vi "Plate Configuration(subVi).vi"(4 "출력 클러스터 2":T1, 5 "all rows":string[][](array[string])=[["", "Well", "Fluor", "Target", "Content", "Sample", "Cq", "SQ"], ["", "A01", "SYBR", "Fos", "Unkn", "Fl1", "23.40", ""], ["", "A02", "SYBR", "Fos", "Unkn", "Fl1", "23.24", ""], ["", "A03", "SYBR", "Fos", "Unkn", "Fl2", "23.55", ""], ["", "A04", "SYBR", "Fos", "Unkn", "Fl2", "23.53", ""], ["", "A05", "SYBR", "Fos", "Unkn", "Fl3", "23.38", ""], ["", "A06", "SYBR", "Fos", "Unkn", "Fl3", "23.50", ""], ["", "A07", "SYBR", "Fos", "Unkn", "Pfl1", "22.43", ""], ["", "A08", "SYBR", "Fos", "Unkn", "Pfl1", "22.94", ""], ["", "A09", "SYBR", "Fos", "Unkn", "Pfl2", "21.10", ""], ["", "A10", "SYBR", "Fos", "Unkn", "Pfl2", "21.46", ""], ["", "A11", "SYBR", "Fos", "Unkn", "Pfl3", "22.49", ""], ["", "A12", "SYBR", "Fos", "Unkn", "Pfl3", "22.89", ""], ["", "B01", "SYBR", "Arc", "Unkn", "Fl1", "32.28", ""], ["", "B02", "SYBR", "Arc", "Unkn", "Fl1", "32.59", ""], ["", "B03", "SYBR", "Arc", "Unkn", "Fl2", "32.93", ""], ["", "B04", "SYBR", "Arc", "Unkn", "Fl2", "32.78", ""], ["", "B05", "SYBR", "Arc", "Unkn", "Fl3", "32.38", ""], ["", "B06", "SYBR", "Arc", "Unkn", "Fl3", "32.35", ""], ["", "B07", "SYBR", "Arc", "Unkn", "Pfl1", "30.44", ""], ["", "B08", "SYBR", "Arc", "Unkn", "Pfl1", "30.58", ""], ["", "B09", "SYBR", "Arc", "Unkn", "Pfl2", "30.07", ""], ["", "B10", "SYBR", "Arc", "Unkn", "Pfl2", "30.20", ""], ["", "B11", "SYBR", "Arc", "Unkn", "Pfl3", "30.38", ""], ["", "B12", "SYBR", "Arc", "Unkn", "Pfl3", "30.04", ""], ["", "C01", "SYBR", "Jun", "Unkn", "Fl1", "25.27", ""], ["", "C02", "SYBR", "Jun", "Unkn", "Fl1", "24.72", ""], ["", "C03", "SYBR", "Jun", "Unkn", "Fl2", "25.47", ""], ["", "C04", "SYBR", "Jun", "Unkn", "Fl2", "25.79", ""], ["", "C05", "SYBR", "Jun", "Unkn", "Fl3", "25.27", ""], ["", "C06", "SYBR", "Jun", "Unkn", "Fl3", "25.52", ""], ["", "C07", "SYBR", "Jun", "Unkn", "Pfl1", "23.53", ""], ["", "C08", "SYBR", "Jun", "Unkn", "Pfl1", "23.37", ""], ["", "C09", "SYBR", "Jun", "Unkn", "Pfl2", "21.29", ""], ["", "C10", "SYBR", "Jun", "Unkn", "Pfl2", "38.35", ""], ["", "C11", "SYBR", "Jun", "Unkn", "Pfl3", "23.20", ""], ["", "C12", "SYBR", "Jun", "Unkn", "Pfl3", "23.23", ""], ["", "D01", "SYBR", "JunB", "Unkn", "Fl1", "26.08", ""], ["", "D02", "SYBR", "JunB", "Unkn", "Fl1", "26.09", ""], ["", "D03", "SYBR", "JunB", "Unkn", "Fl2", "27.02", ""], ["", "D04", "SYBR", "JunB", "Unkn", "Fl2", "27.08", ""], ["", "D05", "SYBR", "JunB", "Unkn", "Fl3", "26.91", ""], ["", "D06", "SYBR", "JunB", "Unkn", "Fl3", "26.93", ""], ["", "D07", "SYBR", "JunB", "Unkn", "Pfl1", "25.32", ""], ["", "D08", "SYBR", "JunB", "Unkn", "Pfl1", "25.12", ""], ["", "D09", "SYBR", "JunB", "Unkn", "Pfl2", "24.28", ""], ["", "D10", "SYBR", "JunB", "Unkn", "Pfl2", "24.21", ""], ["", "D11", "SYBR", "JunB", "Unkn", "Pfl3", "25.01", ""], ["", "D12", "SYBR", "JunB", "Unkn", "Pfl3", "25.38", ""], ["", "E01", "SYBR", "Ctgf", "Unkn", "Fl1", "27.57", ""], ["", "E02", "SYBR", "Ctgf", "Unkn", "Fl1", "27.52", ""], ["", "E03", "SYBR", "Ctgf", "Unkn", "Fl2", "28.24", ""], ["", "E04", "SYBR", "Ctgf", "Unkn", "Fl2", "28.02", ""], ["", "E05", "SYBR", "Ctgf", "Unkn", "Fl3", "28.10", ""], ["", "E06", "SYBR", "Ctgf", "Unkn", "Fl3", "27.90", ""], ["", "E07", "SYBR", "Ctgf", "Unkn", "Pfl1", "25.17", ""], ["", "E08", "SYBR", "Ctgf", "Unkn", "Pfl1", "25.51", ""], ["", "E09", "SYBR", "Ctgf", "Unkn", "Pfl2", "25.49", ""], ["", "E10", "SYBR", "Ctgf", "Unkn", "Pfl2", "25.43", ""], ["", "E11", "SYBR", "Ctgf", "Unkn", "Pfl3", "25.45", ""], ["", "E12", "SYBR", "Ctgf", "Unkn", "Pfl3", "25.45", ""], ["", "F01", "SYBR", "Nr4a1", "Unkn", "Fl1", "25.09", ""], ["", "F02", "SYBR", "Nr4a1", "Unkn", "Fl1", "25.24", ""], ["", "F03", "SYBR", "Nr4a1", "Unkn", "Fl2", "26.15", ""], ["", "F04", "SYBR", "Nr4a1", "Unkn", "Fl2", "26.01", ""], ["", "F05", "SYBR", "Nr4a1", "Unkn", "Fl3", "26.17", ""], ["", "F06", "SYBR", "Nr4a1", "Unkn", "Fl3", "26.29", ""], ["", "F07", "SYBR", "Nr4a1", "Unkn", "Pfl1", "24.23", ""], ["", "F08", "SYBR", "Nr4a1", "Unkn", "Pfl1", "24.26", ""], ["", "F09", "SYBR", "Nr4a1", "Unkn", "Pfl2", "23.05", ""], ["", "F10", "SYBR", "Nr4a1", "Unkn", "Pfl2", "23.08", ""], ["", "F11", "SYBR", "Nr4a1", "Unkn", "Pfl3", "24.02", ""], ["", "F12", "SYBR", "Nr4a1", "Unkn", "Pfl3", "24.04", ""], ["", "G01", "SYBR", "Egr1", "Unkn", "Fl1", "26.85", ""], ["", "G02", "SYBR", "Egr1", "Unkn", "Fl1", "26.59", ""], ["", "G03", "SYBR", "Egr1", "Unkn", "Fl2", "27.75", ""], ["", "G04", "SYBR", "Egr1", "Unkn", "Fl2", "27.76", ""], ["", "G05", "SYBR", "Egr1", "Unkn", "Fl3", "27.92", ""], ["", "G06", "SYBR", "Egr1", "Unkn", "Fl3", "28.27", ""], ["", "G07", "SYBR", "Egr1", "Unkn", "Pfl1", "25.19", ""], ["", "G08", "SYBR", "Egr1", "Unkn", "Pfl1", "24.90", ""], ["", "G09", "SYBR", "Egr1", "Unkn", "Pfl2", "23.36", ""], ["", "G10", "SYBR", "Egr1", "Unkn", "Pfl2", "23.81", ""], ["", "G11", "SYBR", "Egr1", "Unkn", "Pfl3", "24.67", ""], ["", "G12", "SYBR", "Egr1", "Unkn", "Pfl3", "24.81", ""], ["", "H01", "SYBR", "beta-Actin", "Unkn", "Fl1", "22.22", ""], ["", "H02", "SYBR", "beta-Actin", "Unkn", "Fl1", "22.27", ""], ["", "H03", "SYBR", "beta-Actin", "Unkn", "Fl2", "22.94", ""], ["", "H04", "SYBR", "beta-Actin", "Unkn", "Fl2", "22.82", ""], ["", "H05", "SYBR", "beta-Actin", "Unkn", "Fl3", "23.04", ""], ["", "H06", "SYBR", "beta-Actin", "Unkn", "Fl3", "22.72", ""], ["", "H07", "SYBR", "beta-Actin", "Unkn", "Pfl1", "22.09", ""], ["", "H08", "SYBR", "beta-Actin", "Unkn", "Pfl1", "22.09", ""], ["", "H09", "SYBR", "beta-Actin", "Unkn", "Pfl2", "21.57", ""], ["", "H10", "SYBR", "beta-Actin", "Unkn", "Pfl2", "21.16", ""], ["", "H11", "SYBR", "beta-Actin", "Unkn", "Pfl3", "21.80", ""], ["", "H12", "SYBR", "beta-Actin", "Unkn", "Pfl3", "21.93", ""]] caption="모든 행", 6 "RowLabel":T3(array[cluster])=[{"RowNames"="A", "Label"=enum."Target Ch"}, {"RowNames"="B", "Label"=enum."Target Ch"}, {"RowNames"="C", "Label"=enum."Target Ch"}, {"RowNames"="D", "Label"=enum."Target Ch"}, {"RowNames"="E", "Label"=enum."Target Ch"}, {"RowNames"="F", "Label"=enum."Target Ch"}, {"RowNames"="G", "Label"=enum."Target Ch"}, {"RowNames"="H", "Label"=enum."Internal Ctrl"}], 7 "ColLabel":T2(array[cluster])=[{"ColNames"="01", "Label"=enum."11"}, {"ColNames"="02", "Label"=enum."11"}, {"ColNames"="03", "Label"=enum."12"}, {"ColNames"="04", "Label"=enum."12"}, {"ColNames"="05", "Label"=enum."13"}, {"ColNames"="06", "Label"=enum."13"}, {"ColNames"="07", "Label"=enum."13"}, {"ColNames"="08", "Label"=enum."13"}, {"ColNames"="09", "Label"=enum."13"}, {"ColNames"="10", "Label"=enum."13"}, {"ColNames"="11", "Label"=enum."13"}, {"ColNames"="12", "Label"=enum."13"}]) -> (0 "출력 클러스터":T1, 1 "RowHdrs":string[](array[string]), 2 "Internal Ctrl":string[][](array[string]), 3 "Target Gene":string[][][](array[string]))   [LabVIEW 2015]
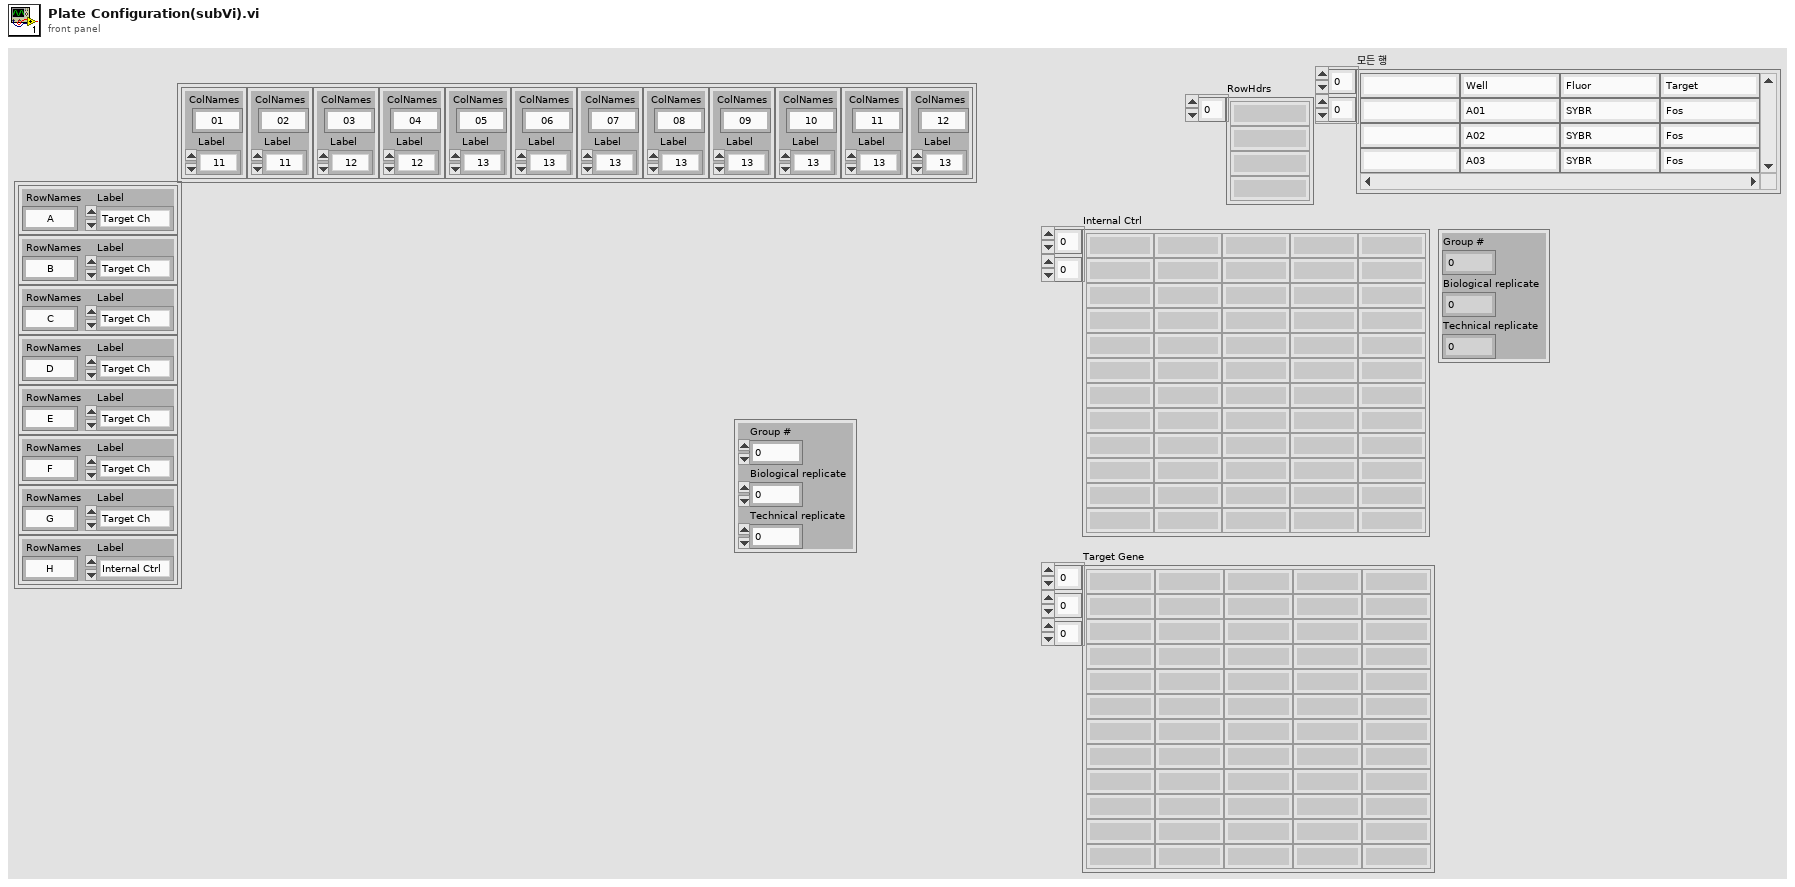
[diagram p1: front panel]
types:
  T1 = cluster{"Group #":dbl, "Biological replicate":dbl, "Technical replicate":dbl}
  T2 = cluster{"ColNames":string, "Label":enum16{"11", "12", "13", "21", "22", "23", "Empty"}}[]
  T3 = cluster{"RowNames":string, "Label":enum16{"Empty Ch", "Target Ch", "Internal Ctrl"}}[]
  T4 = enum16{"11", "12", "13", "21", "22", "23", "Empty"}
  T5 = cluster{"String":string, "String":string, "String":string, "String":string, "String":string}[]
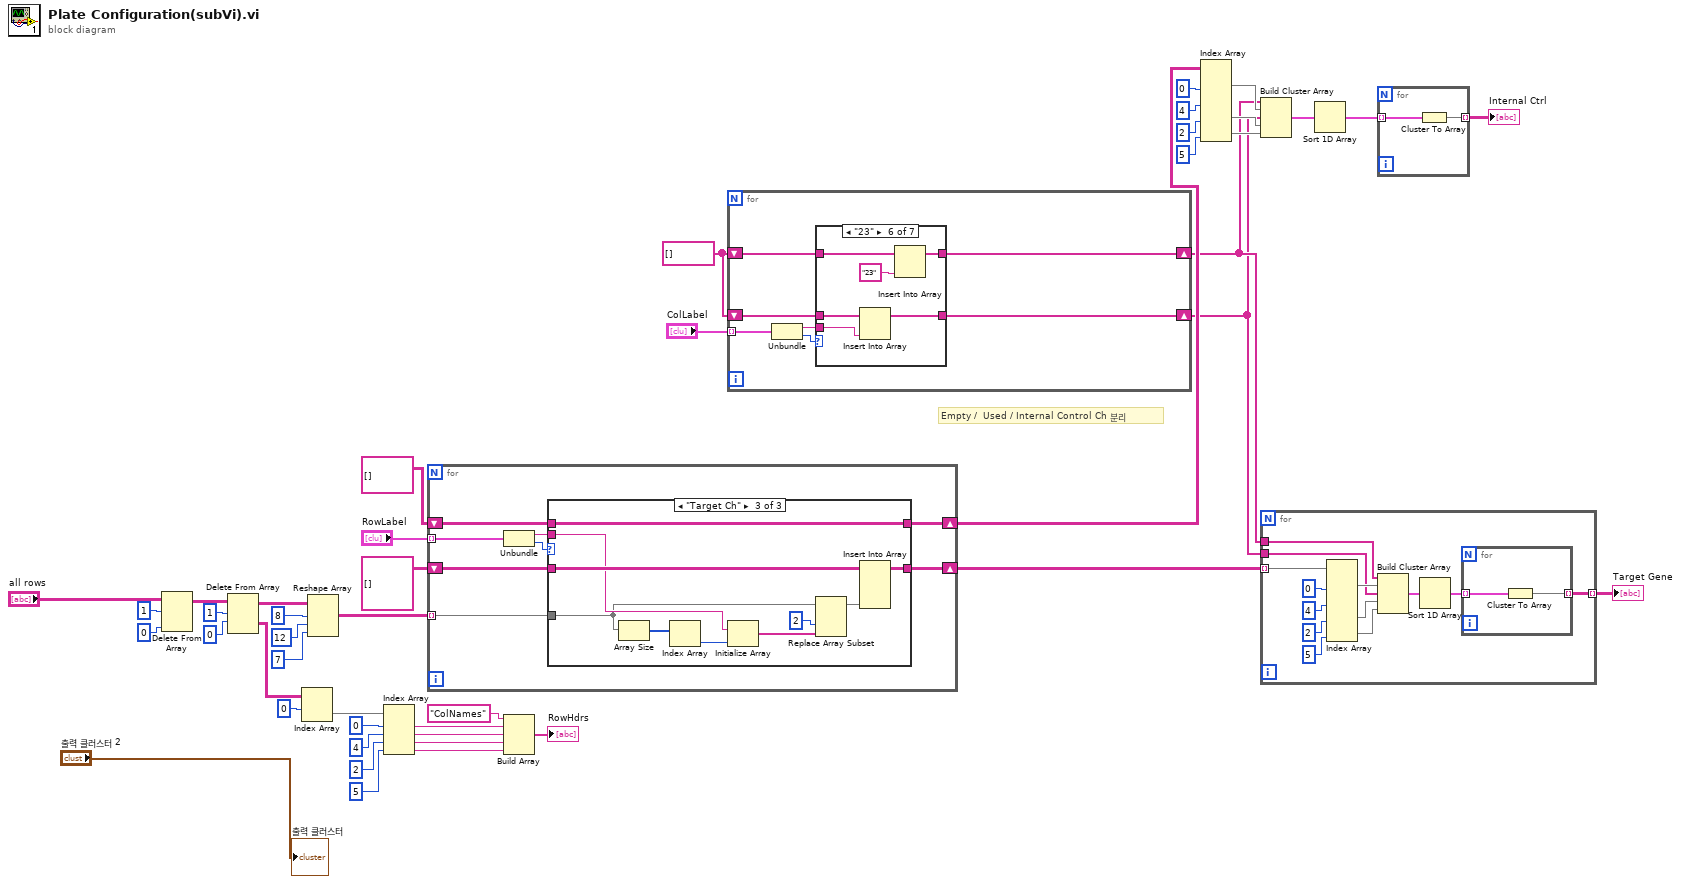
[diagram p0: block diagram]
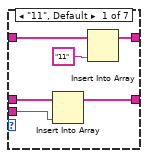
[diagram p2: hidden frame]
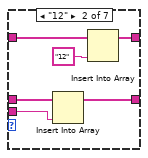
[diagram p3: hidden frame]
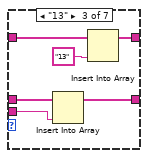
[diagram p4: hidden frame]
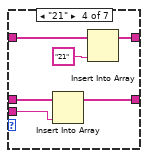
[diagram p5: hidden frame]
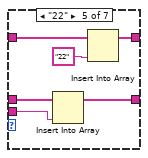
[diagram p6: hidden frame]
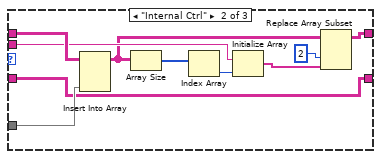
[diagram p9: hidden frame]
diagram:
  w3 = string[] []
  # "Empty /  Used / Internal Control Ch 분리"
  n1 = Delete From Array(array="all rows", length=1 ("길이"), index (col)=0 ("비활성화된 인덱스 (열)")) -> (array with subset deleted=w42:string[][])  [unwired: 1 in, 1 out]
  n2 = Delete From Array(array=w42, length=1 ("길이"), index (row)=0 ("인덱스 (행)")) -> (deleted portion=w17:string[][], array with subset deleted=w36:string[][])  [unwired: 1 in]
  n3 = Index Array(array=w17, index (row)=0 ("인덱스 (행)")) -> (element=w15:string[])  [unwired: 1 in]
  n4 = Reshape Array(w36, 8 ("차원 크기"), 12 ("차원 크기"), 7 ("차원 크기")) -> (w35:string[][][])
  n5 = Index Array(array=w15, index #1=0 ("인덱스"), index #2=4 ("인덱스"), index #3=2 ("인덱스"), index #4=5 ("인덱스")) -> (element #1=w7:string, element #2=w8:string, element #3=w9:string, element #4=w10:string)
  n6 = for {
    tunnel: w35 -> [w51] mode=indexing
    tunnel: "RowLabel" -> [w53] mode=indexing
    shift-right: [w50] -> w31
    shift-left: string[][][] [] -> [w49]
    shift-right: [w47] -> w21
    shift-left: string[][] [] -> [w48]
    n7 = Unbundle(w53) -> ("RowNames"=w46:string, "Label"=w52:enum16{"Empty Ch", "Target Ch", "Internal Ctrl"})
    n8 = case shown="\"Target Ch\"" w52 {
      tunnel: w51 -> [_ w65 w69]
      tunnel: [w55 w63 w73] -> w50
      tunnel: w49 -> [w55 w63 w75]
      tunnel: w48 -> [w54 w64 w74]
      tunnel: [w54 w58 w74] -> w47
      tunnel: w46 -> [_ w62 w70]
      frame "Empty Ch", Default {
      }
      frame "Internal Ctrl" {
        n9 = Insert Into Array(array=w64, new element=w65) -> (w59:string[][])  [unwired: 2 in]
        n10 = Array Size(array=w59) -> (size(s)=w61:i32[])
        n11 = Index Array(array=w61) -> (element=w60:i32)  [unwired: 1 in]
        n12 = Initialize Array(w62, w60) -> (w57:string[])
        n13 = Replace Array Subset(array=w59, new element=w57, index (col)=2 ("비활성화된 인덱스 (열)")) -> (w58:string[][])  [unwired: 1 in]
      }
      frame "Target Ch" {
        n14 = Array Size(array=w69) -> (size(s)=w72:i32[])
        n15 = Index Array(array=w72) -> (element=w71:i32)  [unwired: 1 in]
        n16 = Initialize Array(w70, w71) -> (w68:string[])
        n17 = Replace Array Subset(array=w69, new element=w68, index (col)=2 ("비활성화된 인덱스 (열)")) -> (w66:string[][])  [unwired: 1 in]
        n18 = Insert Into Array(array=w75, new element=w66) -> (w73:string[][][])  [unwired: 3 in]
      }
    }
  }
  n19 = Build Array("ColNames" ("원소"), w7, w8, w9, w10) -> (→"RowHdrs":string[])
  n20 = for {
    tunnel: "ColLabel" -> [w82] mode=indexing
    shift-right: [w79] -> w4
    shift-left: w3 -> [w80]
    shift-right: [w77] -> w2
    shift-left: w3 -> [w76]
    n21 = Unbundle(w82) -> ("ColNames"=w78:string, "Label"=w81:T4)
    n22 = case shown="\"23\"" w81 {
      tunnel: [w87 w92 w99 w105 w111 w117 w120] -> w79
      tunnel: w80 -> [w88 w93 w100 w106 w112 w116 w120]
      tunnel: w78 -> [w83 w89 w97 w101 w107 w113 _]
      tunnel: [w84 w91 w96 w102 w108 w115 w119] -> w77
      tunnel: w76 -> [w85 w90 w95 w103 w109 w114 w119]
      frame "11", Default {
        n23 = Insert Into Array(array=w85, new element=w83) -> (w84:string[])  [unwired: 1 in]
        n24 = Insert Into Array(array=w88, new element="11") -> (w87:string[])  [unwired: 1 in]
      }
      frame "12" {
        n25 = Insert Into Array(array=w90, new element=w89) -> (w91:string[])  [unwired: 1 in]
        n26 = Insert Into Array(array=w93, new element="12") -> (w92:string[])  [unwired: 1 in]
      }
      frame "13" {
        n27 = Insert Into Array(array=w95, new element=w97) -> (w96:string[])  [unwired: 1 in]
        n28 = Insert Into Array(array=w100, new element="13") -> (w99:string[])  [unwired: 1 in]
      }
      frame "21" {
        n29 = Insert Into Array(array=w103, new element=w101) -> (w102:string[])  [unwired: 1 in]
        n30 = Insert Into Array(array=w106, new element="21") -> (w105:string[])  [unwired: 1 in]
      }
      frame "22" {
        n31 = Insert Into Array(array=w109, new element=w107) -> (w108:string[])  [unwired: 1 in]
        n32 = Insert Into Array(array=w112, new element="22") -> (w111:string[])  [unwired: 1 in]
      }
      frame "23" {
        n33 = Insert Into Array(array=w114, new element=w113) -> (w115:string[])  [unwired: 1 in]
        n34 = Insert Into Array(array=w116, new element="23") -> (w117:string[])  [unwired: 1 in]
      }
      frame "Empty" {
      }
    }
  }
  n35 = Index Array(array=w21, index (col) #1=0 ("비활성화된 인덱스 (열)"), index (col) #2=4 ("인덱스 (열)"), index (col) #3=2 ("인덱스 (열)"), index (col) #4=5 ("인덱스 (열)")) -> (element #1=w26:string[], element #3=w27:string[], element #4=w28:string[])  [unwired: 4 in, 1 out]
  n36 = Build Cluster Array(w4, w26, w2, w27, w28) -> (w29:T5)
  n37 = for {
    tunnel: w31 -> [w133] mode=indexing
    tunnel: [w123] -> w19 mode=indexing
    tunnel: w4 -> [w122]
    tunnel: w2 -> [w121]
    n38 = Index Array(array=w133, index (col) #1=0 ("비활성화된 인덱스 (열)"), index (col) #2=4 ("인덱스 (열)"), index (col) #3=2 ("인덱스 (열)"), index (col) #4=5 ("인덱스 (열)")) -> (element #1=w128:string[], element #3=w127:string[], element #4=w126:string[])  [unwired: 4 in, 1 out]
    n39 = Build Cluster Array(w122, w128, w121, w127, w126) -> (w125:T5)
    n40 = Sort 1D Array(array=w125) -> (sorted array=w124:T5)
    n41 = for {
      tunnel: w124 -> [w135] mode=indexing
      tunnel: [w134] -> w123 mode=indexing
      n42 = Cluster To Array(cluster=w135) -> (array=w134:string[])
    }
  }
  "Target Gene" <- w19
  n43 = Sort 1D Array(array=w29) -> (sorted array=w30:T5)
  n44 = for {
    tunnel: w30 -> [w137] mode=indexing
    tunnel: [w136] -> w20 mode=indexing
    n45 = Cluster To Array(cluster=w137) -> (array=w136:string[])
  }
  "Internal Ctrl" <- w20
  "출력 클러스터" <- "출력 클러스터 2"
